vi "PlayingState.vi"(8 "error in (no error)":errorcluster, 11 "PlayingState in":refnum<class "PlayingState.lvclass">) -> (0 "error out":errorcluster, 3 "PlayingState out":refnum<class "PlayingState.lvclass">)   [LabVIEW 2017, in "PlayingState.lvclass"]
uses:
  PlayingState.lvclass
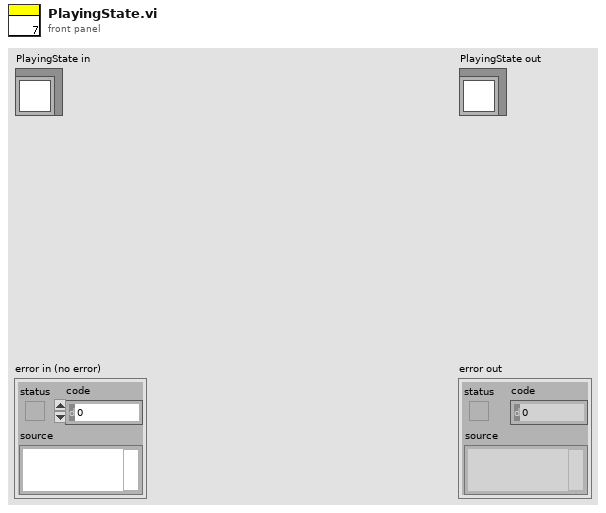
[diagram p1: front panel]
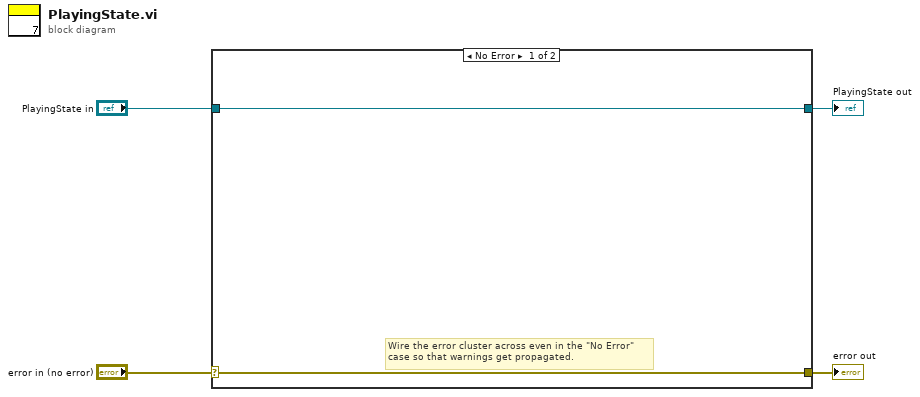
[diagram p0: block diagram]
diagram:
  n1 = case shown="No Error" "error in (no error)" {
    selector: "error in (no error)" -> [w5 w8]
    tunnel: [w5 w8] -> w3
    tunnel: [w6 w7] -> w1
    tunnel: "PlayingState in" -> [w6 w7]
    frame No Error {
      # "Wire the error cluster across even in the \"No Error\"\ncase so that warnings get propagated."
    }
    frame Error {
    }
  }
  "error out" <- w3
  "PlayingState out" <- w1
